vi "Construct Terminal Caption Binding.vi"(10 "Ctl Refnum":refnum<vi>) -> (0 "error out":errorcluster, 3 "TerminalCaptionBinding":refnum<class "TerminalCaptionBinding.lvclass">)   [LabVIEW 2020, in "MVA Framework.lvlib" / "TerminalCaptionBinding.lvclass"]
doc: "构建终端标题绑定"
uses:
  TerminalCaptionBinding.lvclass
  TerminalPropertyBinding/TerminalPropertyBinding.lvclass/TerminalPropertyBinding.ctl
  <vilib>/Utility/error.llb/Error Cluster From Error Code.vi
  <vilib>/ErrorRing/Error Ring.xnode
  TerminalPropertyBinding/TerminalPropertyBinding.lvclass
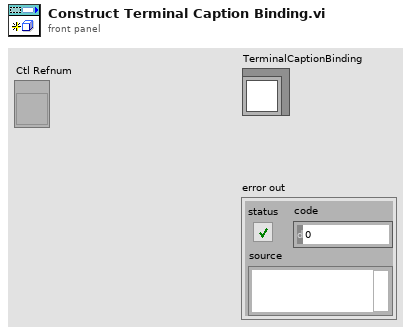
[diagram p1: front panel]
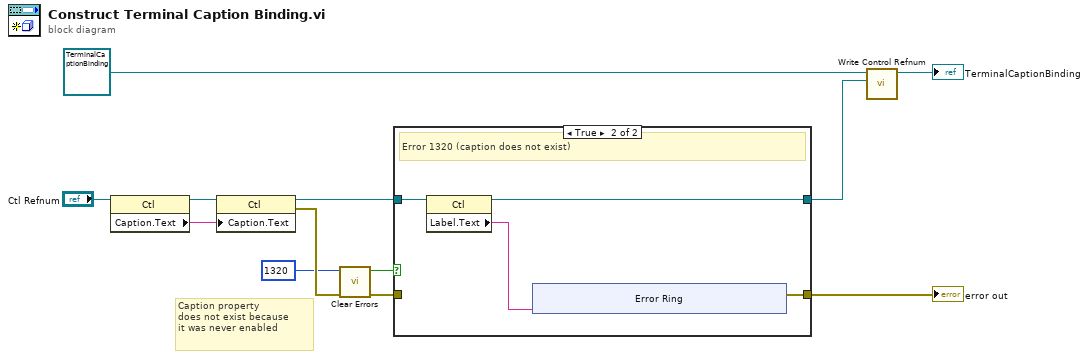
[diagram p0: block diagram]
diagram:
  # "Caption property\ndoes not exist because\nit was never enabled"
  n1 = property class="Ctl"(reference="Ctl Refnum") -> (reference out=w4:refnum<vi>, "Caption.Text"=w3:string)  [unwired: 1 in, 1 out]
  n2 = property class="Ctl"(reference=w4, "Caption.Text"=w3) -> (reference out=w10:refnum<vi>, error out=w7:errorcluster)  [unwired: 1 in]
  n3 = call <vilib>:"Clear Errors.vi"("error in (no error)"=w7, "specific error code to clear (0: all)"=1320) -> ("error out"=w6:errorcluster, "specific error cleared?"=w8:bool)  [unwired: 4 in]
  n4 = case shown="True" w8 {
    tunnel: [w13 w18] -> w11
    tunnel: w10 -> [w14 w17]
    tunnel: [w14 w16] -> w9
    tunnel: w6 -> [w13 _]
    frame False {
    }
    frame True {
      # "Error 1320 (caption does not exist)"
      n5 = property class="Ctl"(reference=w17) -> (reference out=w16:refnum<vi>, "Label.Text"=w15:string)  [unwired: 1 in, 1 out]
      n6 = xnode "Error Ring"("parameter 0"=w15) -> ("error out"=w18:errorcluster)
    }
  }
  "error out" <- w11
  n7 = call "Write Control Refnum.vi"("Ctl Refnum"=w9, "TerminalReference in"=refnum<class "TerminalCaptionBinding.lvclass"> refnum ("ControlCaptionBinding")) -> ("TerminalReferenceBinding Out"=→"TerminalCaptionBinding":refnum<class "TerminalCaptionBinding.lvclass">)  [unwired: 9 in]
